vi "GraphForces.vi"(8 "Tot envir":dbl[](array[numeric]), 9 "D_L":dbl[](array[numeric]), 10 "D_NL":dbl[](array[numeric]), 11 "Umbilical":dbl[](array[numeric])) -> ()   [LabVIEW 2014]
panel:
  out "Total heave":cluster{"Y":dbl[], "Y":dbl[]}[](graph)
  out "Total sway":cluster{"Y":dbl[], "Y":dbl[]}[](graph)
  out "Total surge":cluster{"Y":dbl[], "Y":dbl[]}[](graph)
  out "D_L heave":cluster{"Y":dbl[], "Y":dbl[]}[](graph)
  out "D_L sway":cluster{"Y":dbl[], "Y":dbl[]}[](graph)
  out "D_L surge":cluster{"Y":dbl[], "Y":dbl[]}[](graph)
  out "D_NL heave":cluster{"Y":dbl[], "Y":dbl[]}[](graph)
  out "D_NL sway":cluster{"Y":dbl[], "Y":dbl[]}[](graph)
  out "D_NL surge":cluster{"Y":dbl[], "Y":dbl[]}[](graph)
  out "Umbilical pitch":cluster{"Y":dbl[], "Y":dbl[]}[](graph)
  out "Umbilical roll":cluster{"Y":dbl[], "Y":dbl[]}[](graph)
  out "Umbilical sway":cluster{"Y":dbl[], "Y":dbl[]}[](graph)
  out "Umbilical surge":cluster{"Y":dbl[], "Y":dbl[]}[](graph)
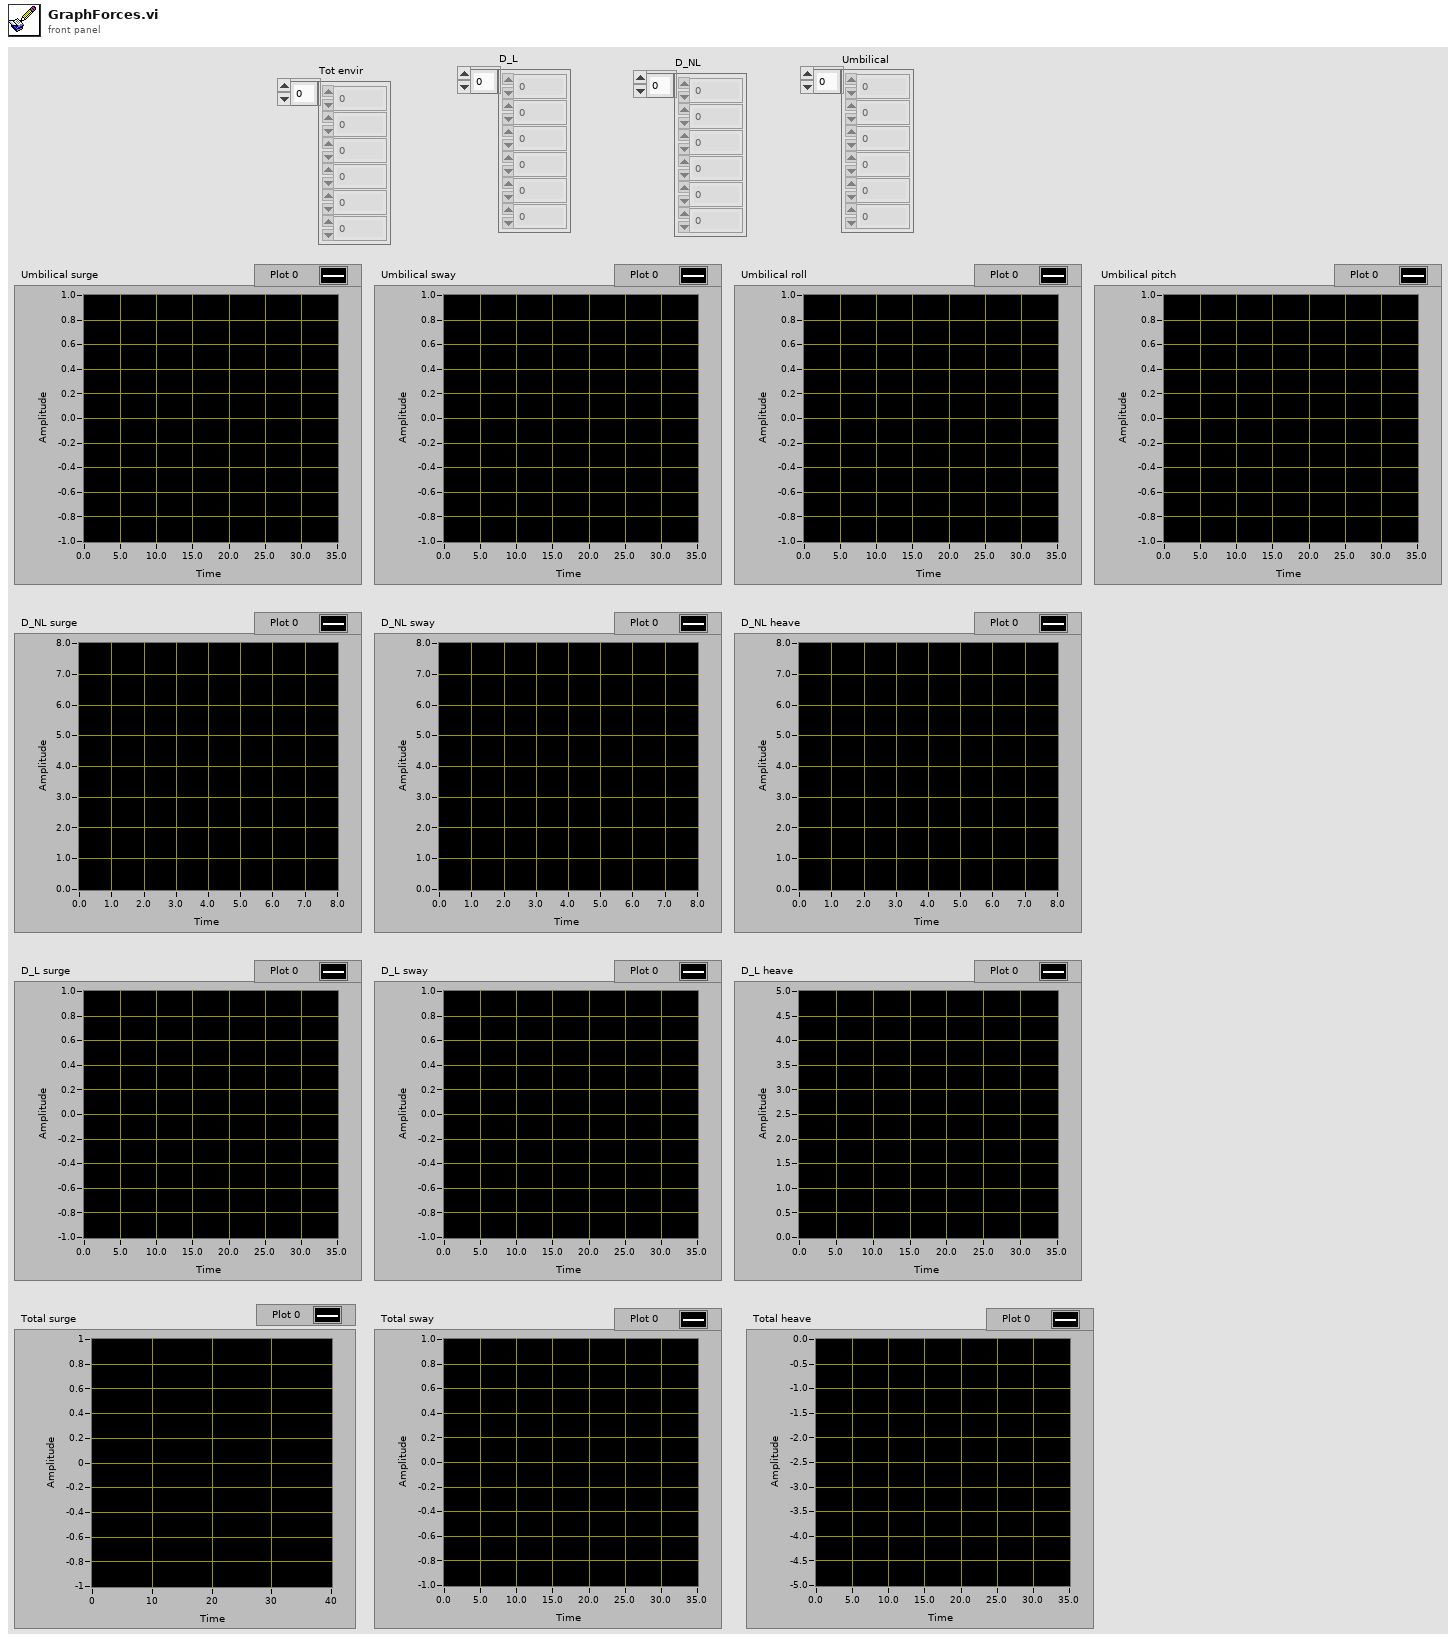
[diagram p1: front panel]
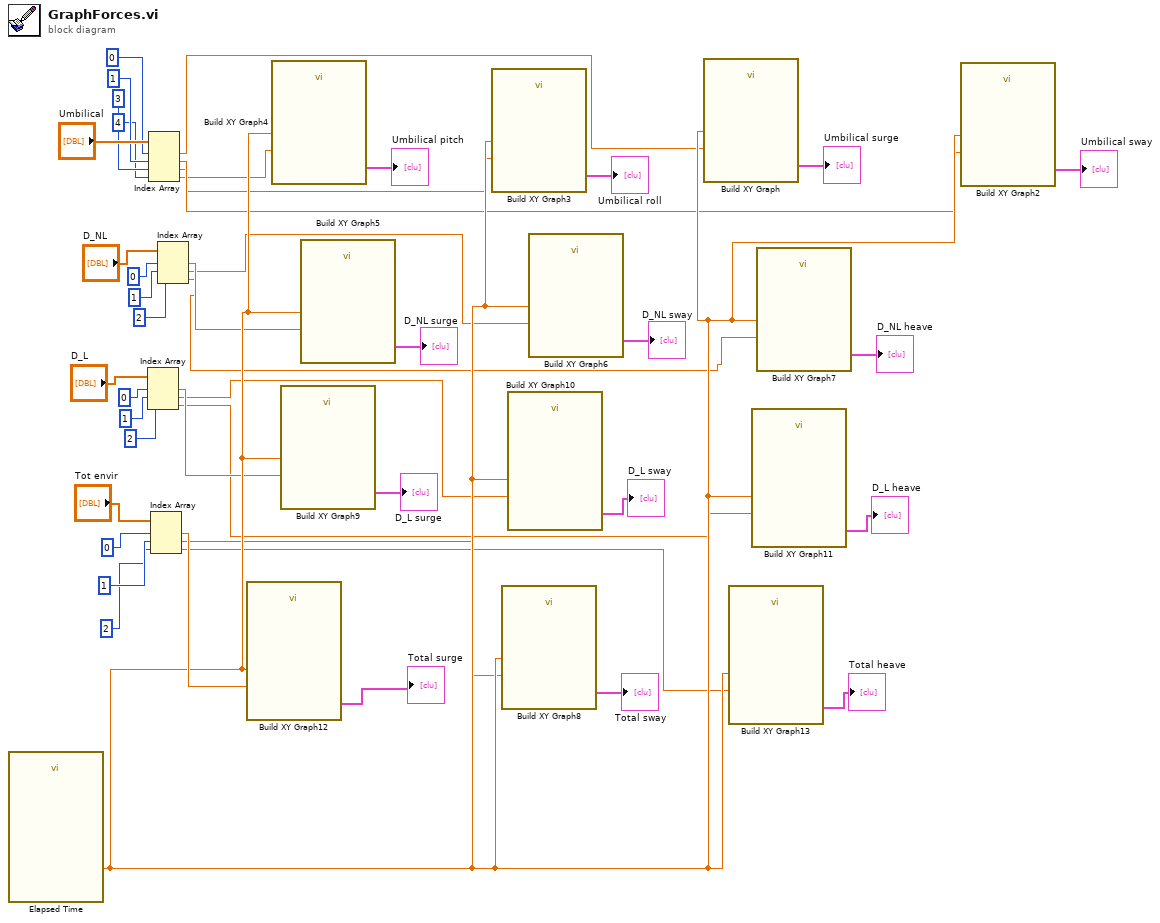
[diagram p0: block diagram]
diagram:
  n1 = call "Elapsed Time"() -> ("Elapsed Time (s)"=w28:dbl)  [unwired: 12 in, 7 out]
  n2 = Index Array(array="D_L", index #1=0, index #2=1, index #3=2) -> (element #1=w17:dbl, element #2=w16:dbl, element #3=w15:dbl)
  n3 = Index Array(array="Umbilical", index #1=0, index #2=1, index #3=3, index #4=4) -> (element #1=w7:dbl, element #2=w6:dbl, element #3=w5:dbl, element #4=w4:dbl)
  n4 = Index Array(array="Tot envir", index #1=0, index #2=1, index #3=2) -> (element #1=w29:dbl, element #2=w25:dbl, element #3=w24:dbl)
  n5 = Index Array(array="D_NL", index #1=0, index #2=1, index #3=2) -> (element #1=w3:dbl, element #2=w2:dbl, element #3=w1:dbl)
  n6 = call "Build XY Graph12"("Y Input"=w29, "X Input"=w28) -> ("XY Graph"=→"Total surge":cluster{"Y":dbl[], "Y":dbl[]}[])  [unwired: 3 in, 6 out]
  n7 = call "Build XY Graph4"("Y Input"=w4, "X Input"=w28) -> ("XY Graph"=→"Umbilical pitch":cluster{"Y":dbl[], "Y":dbl[]}[])  [unwired: 3 in, 6 out]
  n8 = call "Build XY Graph9"("Y Input"=w17, "X Input"=w28) -> ("XY Graph"=→"D_L surge":cluster{"Y":dbl[], "Y":dbl[]}[])  [unwired: 3 in, 6 out]
  n9 = call "Build XY Graph5"("Y Input"=w3, "X Input"=w28) -> ("XY Graph"=→"D_NL surge":cluster{"Y":dbl[], "Y":dbl[]}[])  [unwired: 3 in, 6 out]
  n10 = call "Build XY Graph3"("Y Input"=w5, "X Input"=w28) -> ("XY Graph"=→"Umbilical roll":cluster{"Y":dbl[], "Y":dbl[]}[])  [unwired: 3 in, 6 out]
  n11 = call "Build XY Graph8"("Y Input"=w25, "X Input"=w28) -> ("XY Graph"=→"Total sway":cluster{"Y":dbl[], "Y":dbl[]}[])  [unwired: 3 in, 6 out]
  n12 = call "Build XY Graph10"("Y Input"=w16, "X Input"=w28) -> ("XY Graph"=→"D_L sway":cluster{"Y":dbl[], "Y":dbl[]}[])  [unwired: 3 in, 6 out]
  n13 = call "Build XY Graph6"("Y Input"=w2, "X Input"=w28) -> ("XY Graph"=→"D_NL sway":cluster{"Y":dbl[], "Y":dbl[]}[])  [unwired: 3 in, 6 out]
  n14 = call "Build XY Graph"("Y Input"=w7, "X Input"=w28) -> ("XY Graph"=→"Umbilical surge":cluster{"Y":dbl[], "Y":dbl[]}[])  [unwired: 3 in, 6 out]
  n15 = call "Build XY Graph13"("Y Input"=w24, "X Input"=w28) -> ("XY Graph"=→"Total heave":cluster{"Y":dbl[], "Y":dbl[]}[])  [unwired: 3 in, 6 out]
  n16 = call "Build XY Graph11"("Y Input"=w15, "X Input"=w28) -> ("XY Graph"=→"D_L heave":cluster{"Y":dbl[], "Y":dbl[]}[])  [unwired: 3 in, 6 out]
  n17 = call "Build XY Graph7"("Y Input"=w1, "X Input"=w28) -> ("XY Graph"=→"D_NL heave":cluster{"Y":dbl[], "Y":dbl[]}[])  [unwired: 3 in, 6 out]
  n18 = call "Build XY Graph2"("Y Input"=w6, "X Input"=w28) -> ("XY Graph"=→"Umbilical sway":cluster{"Y":dbl[], "Y":dbl[]}[])  [unwired: 3 in, 6 out]
